vi "Add Children to Tree.vi"(8 "error in (no error)":errorcluster, 9 "Parent Tag":string, 10 "Tree Manager in":refnum<class "Tree Manager.lvclass">, 11 "Data Item in":refnum<class "Data Item.lvclass">) -> (0 "error out":errorcluster, 2 "Tree Manager out":refnum<class "Tree Manager.lvclass">, 3 "Data Item out":refnum<class "Data Item.lvclass">)   [LabVIEW 2020, in "VILab.lvlib" / "Data Item.lvclass"]
uses:
  Data Item.lvclass
  Tree Manager/Tree Manager.lvclass
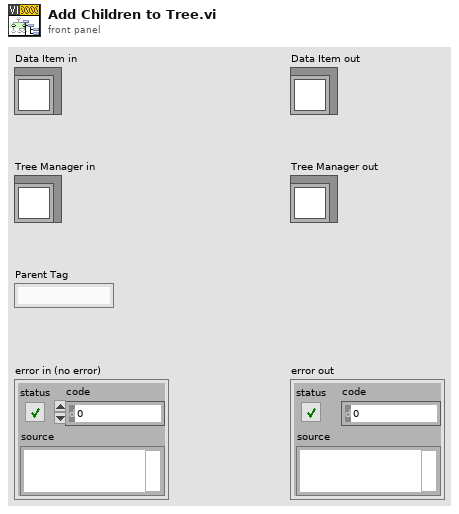
[diagram p1: front panel]
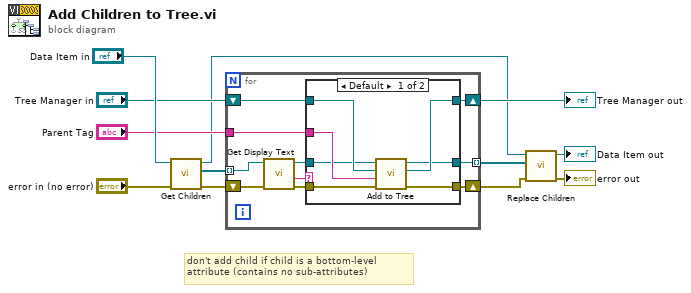
[diagram p0: block diagram]
diagram:
  # "don't add child if child is a bottom-level attribute (contains no sub-attributes)"
  n1 = call-dynamic "Get Children.vi"("error in (no error)"="error in (no error)", "Data Item in"="Data Item in") -> ("error out"=w11:errorcluster, "Children"=w12:refnum<class "Data Item.lvclass">[], "Data Item out"=w1:refnum<class "Data Item.lvclass">)  [unwired: 7 in]
  n2 = for {
    shift-right: [w19] -> w4
    shift-left: "Tree Manager in" -> [w21]
    shift-right: [w20] -> w7
    shift-left: w11 -> [w14]
    tunnel: w12 -> [w22] mode=indexing
    tunnel: "Parent Tag" -> [w18]
    tunnel: [w17] -> w5 mode=indexing
    n3 = call-dynamic "Get Display Text.vi"("error in (no error)"=w14, "Data Item in"=w22) -> ("error out"=w13:errorcluster, "Detail Text"=w15:string, "Data Item out"=w16:refnum<class "Data Item.lvclass">)  [unwired: 6 in, 1 out]
    n4 = case shown="Default" w15 {
      tunnel: w21 -> [w29 w32]
      tunnel: w13 -> [w28 w30]
      tunnel: [w27 w30] -> w20
      tunnel: [w26 w32] -> w19
      tunnel: w18 -> [w25 _]
      tunnel: [w24 w31] -> w17
      tunnel: w16 -> [w23 w31]
      frame Default {
        n5 = call-dynamic "Add to Tree.vi"("error in (no error)"=w28, "Parent Tag"=w25, "Tree Manager in"=w29, "Data Item in"=w23) -> ("error out"=w27:errorcluster, "Tree Manager out"=w26:refnum<class "Tree Manager.lvclass">, "Data Item out"=w24:refnum<class "Data Item.lvclass">)  [unwired: 5 in]
      }
      frame "" {
      }
    }
  }
  "Tree Manager out" <- w4
  n6 = call-dynamic "Replace Children.vi"("error in (no error)"=w7, "New Children"=w5, "Data Item in"=w1) -> ("error out"=→"error out":errorcluster, "Data Item out"=→"Data Item out":refnum<class "Data Item.lvclass">)  [unwired: 7 in]
